vi "AcquireWaveformsFpga.vi"(8 "error in (no error)":errorcluster, 11 "923x Acquisition Config":T1={"NumberOfModules"=0, "Dynamic FPGA VI Ref"=refnum, "KeyphasorX3"=[], "FixedSizeX24"={"EnabledChannels"=[], "Sensitivity"=[], "InputConfig"=[]}, "SamplingInfo"={"Number of Channels"=4, "Sampling Rate"=4.0, "Channels"=[], "Units"=[]}, "BlockSize (sec)"=0.0, "Samples To Read (per chan)"=0, "RunningAcquisitionLength"=0.0, "Settling Time"=0.0, "Waveform Groups"=[], "Acquisition Block Number"=0, "Device Name"="", "ValidConfig"=FALSE} {"FixedSizeX24"."InputConfig" items=["AC Coupled", "DC Coupled", "IEPE AC Coupled"]}) -> (0 "error out":errorcluster, 3 "Waveforms":waveform(sgl)[](array[waveform]), 4 "Data Rate [S/s]":u32)   [LabVIEW 2015]
uses:
  <vilib>/addons/InsightCM/Devices/Shared/AcquireBaseLoop/controls/Configuration.ctl
  <vilib>/addons/InsightCM/Devices/Shared/AcquireBaseLoop/controls/TachometerConfig.ctl
  <vilib>/addons/InsightCM/Devices/Shared/AcquireBaseLoop/controls/FixedSizeArrays.ctl
  <vilib>/LabVIEW Targets/FPGA/cRIO/shared/nicrio_ModuleControls/nicrio_cRIO-9232_ConfigModeRing.ctl
  <vilib>/addons/InsightCM/Devices/Shared/cRIOWfmAcq/subVIs/RIO Wfm Cust Ctrls/rwfm_SamplingInfo.ctl
  <vilib>/addons/InsightCM/Devices/Shared/AcquireBaseLoop/controls/Group.ctl
  <vilib>/addons/InsightCM/Devices/Shared/AcquireBaseLoop/controls/Channel.ctl
  <vilib>/addons/InsightCM/Utilities/ChannelStatus/controls/RangeParams.ctl
  <vilib>/addons/InsightCM/Devices/Shared/cRIOWfmAcq/cRIOWfmLib.lvlib
  <vilib>/addons/InsightCM/Devices/Shared/AcquireBaseLoop/FpgaAcquisition923x.lvlib
  <vilib>/addons/InsightCM/Utilities/ChannelStatus/ChannelStatus.lvlib
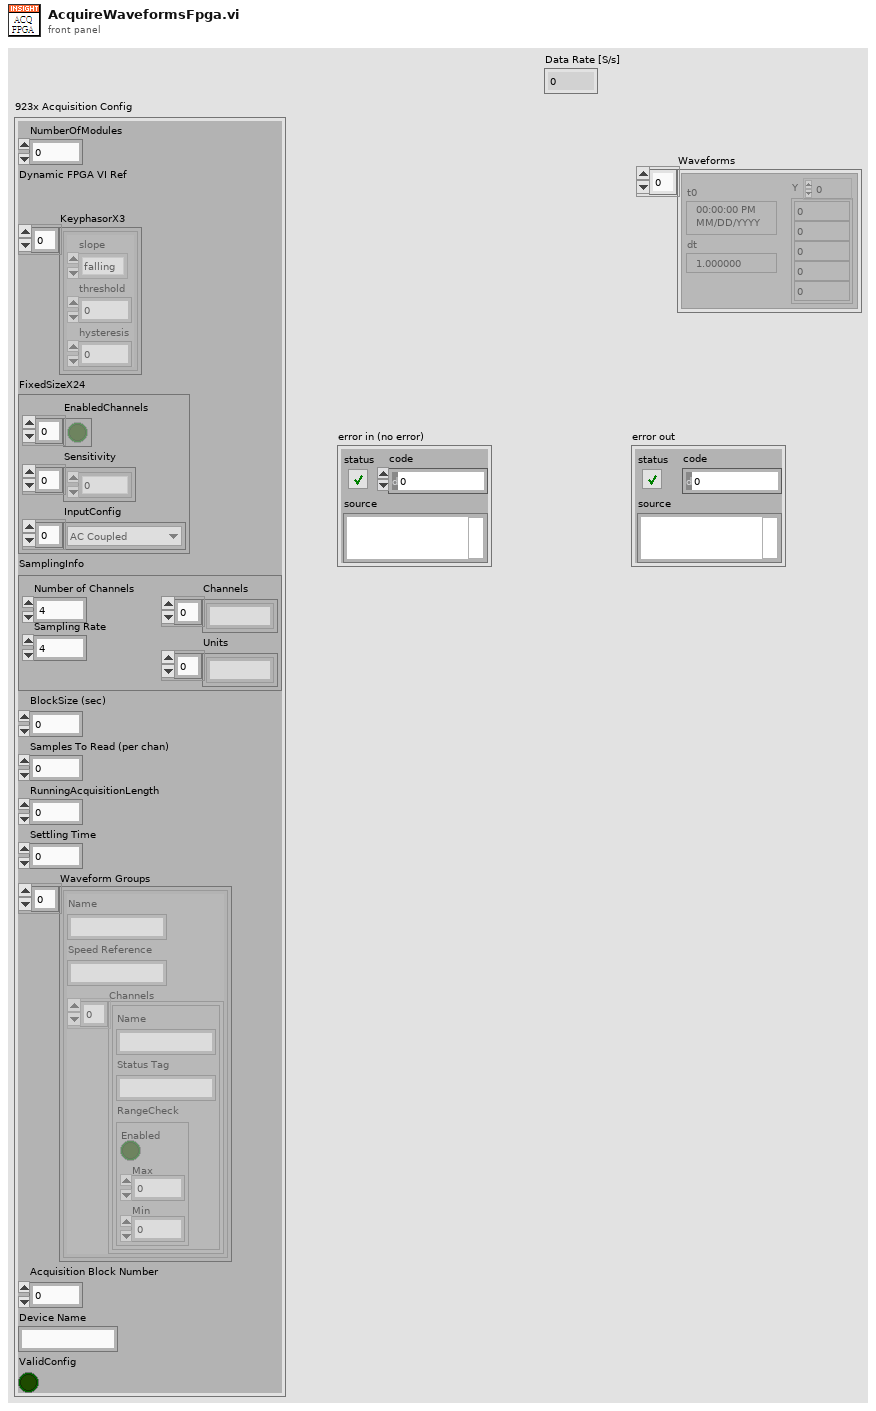
[diagram p1: front panel]
types:
  T1 = typedef "FpgaAcquisition923x.lvlib/Configuration.ctl" = cluster{"NumberOfModules":i16, "Dynamic FPGA VI Ref":refnum<k20>, "KeyphasorX3":T2[], "FixedSizeX24":T3, "SamplingInfo":T5, "BlockSize (sec)":dbl, "Samples To Read (per chan)":i32, "RunningAcquisitionLength":dbl, "Settling Time":dbl, "Waveform Groups":T6[], "Acquisition Block Number":i32, "Device Name":string, "ValidConfig":bool}
  T2 = typedef "FpgaAcquisition923x.lvlib/TachometerConfig.ctl" = cluster{"slope":enum16{"falling", "rising"}, "threshold":dbl, "hysteresis":dbl}
  T3 = typedef "FpgaAcquisition923x.lvlib/FixedSizeArrays.ctl" = cluster{"EnabledChannels":bool[], "Sensitivity":dbl[], "InputConfig":T4[]}
  T4 = typedef "nicrio_cRIO-9232_ConfigModeRing.ctl" = u8
  T5 = typedef "cRIOWfmLib.lvlib/rwfm_SamplingInfo.ctl" = cluster{"Number of Channels":i32, "Sampling Rate":dbl, "Channels":string[], "Units":string[]}
  T6 = typedef "FpgaAcquisition923x.lvlib/Group.ctl" = cluster{"Name":string, "Speed Reference":string, "Channels":T7[]}
  T7 = typedef "FpgaAcquisition923x.lvlib/Channel.ctl" = cluster{"Name":string, "Status Tag":string, "RangeCheck":T8}
  T8 = typedef "ChannelStatus.lvlib/RangeParams.ctl" = cluster{"Enabled":bool, "Max":dbl, "Min":dbl}
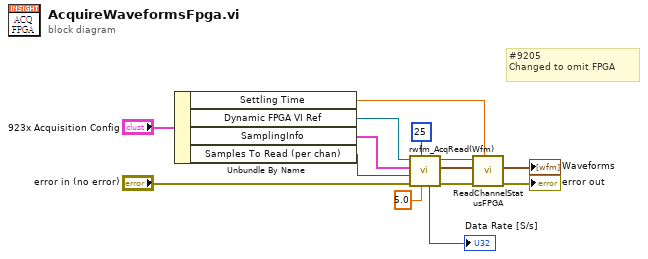
[diagram p0: block diagram]
diagram:
  # "#9205\nChanged to omit FPGA"
  n1 = Unbundle By Name("923x Acquisition Config") -> ("Settling Time"=w5:dbl, "Dynamic FPGA VI Ref"=w4:refnum<k20>, "SamplingInfo"=w3:T5, "Samples To Read (per chan)"=w2:i32)
  n2 = call <vilib>:"rwfm_AcqRead(Wfm).vi"("Timeout (s)"=5.0, "Poll Time (ms)"=u32 25, "error in"="error in (no error)", "Samps Read per Chan"=w2, "Sampling Info"=w3, "Dynamic FPGA VI Reference"=w4) -> ("error out"=w12:errorcluster, "Wfm Data"=w11:waveform(sgl)[], "Dynamic FPGA VI Reference"=w10:refnum<k20>, "Data Rate [S/s]"=→"Data Rate [S/s]":u32)  [unwired: 2 out]
  n3 = call "ReadChannelStatusFPGA.vi"("IEPE settling blocks"=w5, "error in"=w12, "Wfm Data"=w11, "Dynamic FPGA VI Reference"=w10) -> ("error out"=→"error out":errorcluster, "Wfm Data"=→"Waveforms":waveform(sgl)[])  [unwired: 5 in, 1 out]
